vi "NV40.vi"(4 "Position":dbl, 5 "error in (no error)":errorcluster, 6 "Timeout":u32=100, 7 "VISA resource name":refnum<visa-resource-name>, 8 "Command":T1(ring)) -> (0 "error out":errorcluster, 3 "Position out":dbl)   [LabVIEW 2015]
uses:
  <vilib>/Instr/_visa.llb/VISA Open Access Mode.ctl
  <vilib>/Instr/_visa.llb/VISA Configure Serial Port (Instr).vi
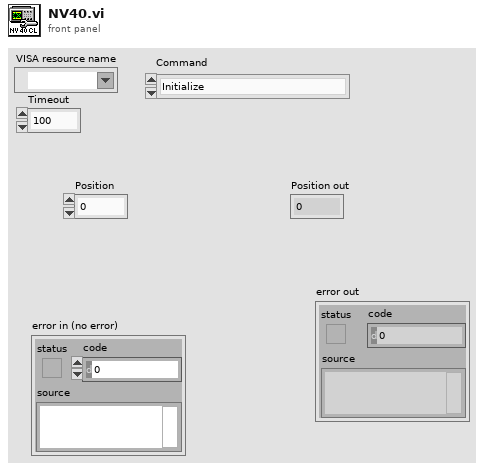
[diagram p1: front panel]
types:
  T1 = enum16{"Initialize", "Close", "Set position", "Get position", "Closed loop on", "Closed loop off", "Remote control on", "Remote control off"}
  T2 = typedef "VISA Open Access Mode.ctl" = u32
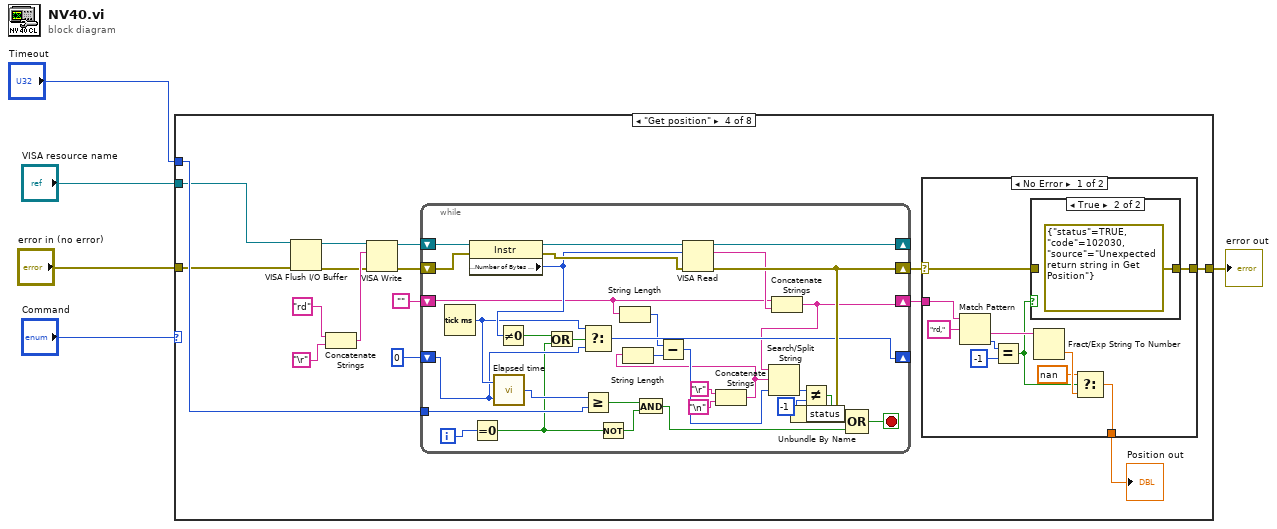
[diagram p0: block diagram]
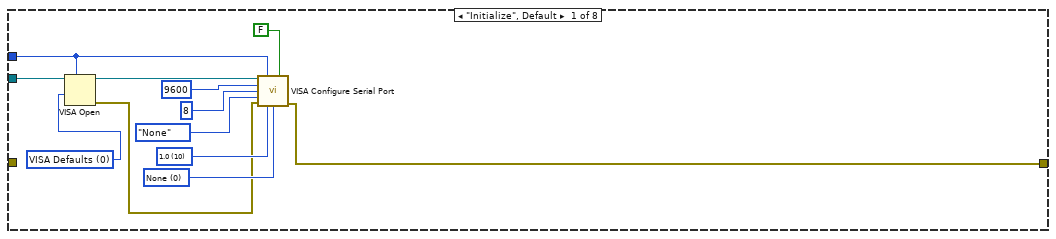
[diagram p2: hidden frame]
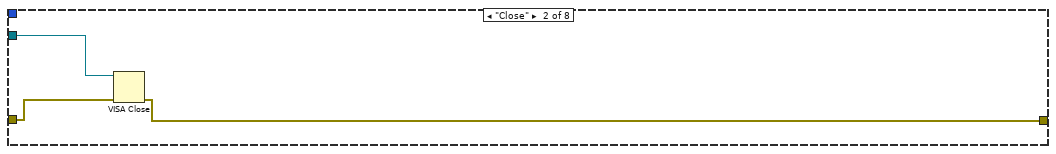
[diagram p3: hidden frame]
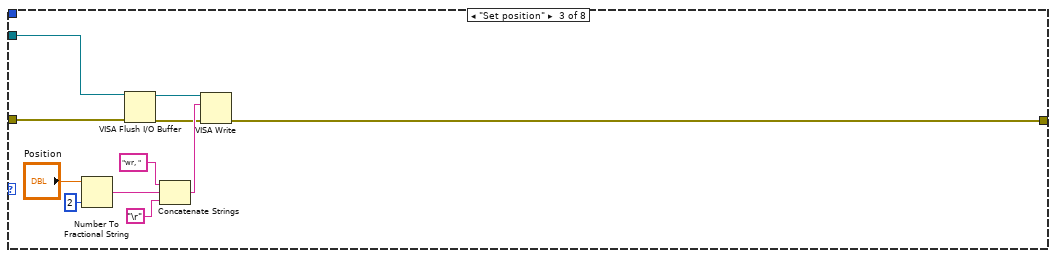
[diagram p4: hidden frame]
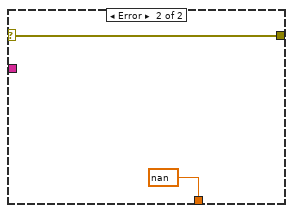
[diagram p6: hidden frame]
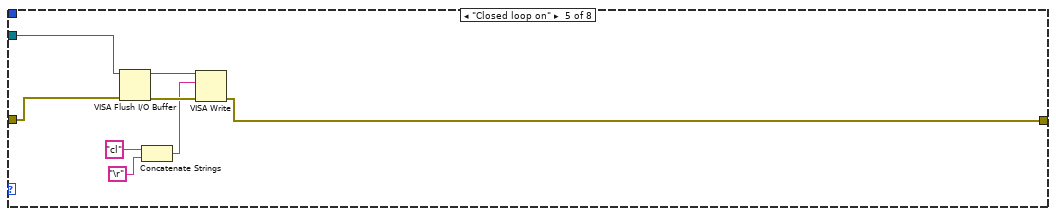
[diagram p7: hidden frame]
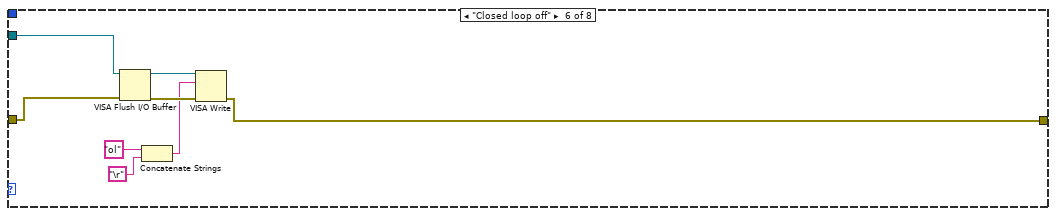
[diagram p8: hidden frame]
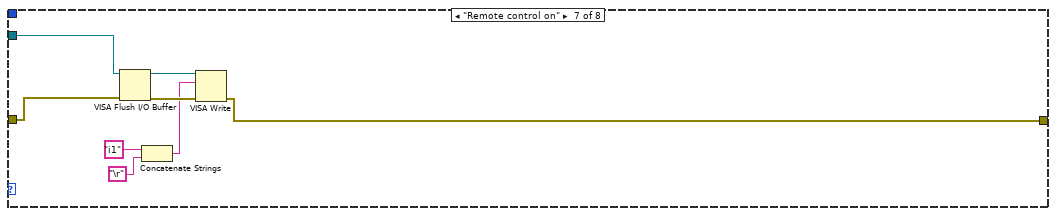
[diagram p9: hidden frame]
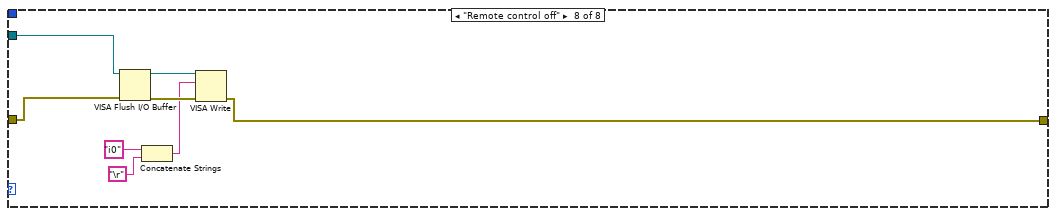
[diagram p10: hidden frame]
diagram:
  n1 = case shown="\"Get position\"" "Command" {
    tunnel: [w6 w18 w25 w33 w99 w107 w115 w123] -> w5
    tunnel: "Timeout" -> [w9 _ _ w39 _ _ _ _]
    tunnel: "VISA resource name" -> [w11 w20 w27 w38 w101 w109 w117 w125]
    tunnel: "error in (no error)" -> [_ w19 w26 w37 w100 w108 w116 w124]
    frame "Initialize", Default {
      w8 = T2 0 items=["VISA Defaults"=0, "Exclusive Lock"=1, "Load Configured Settings"=4] ("Access Mode")
      w12 = u16 0 items=["None", "XON/XOFF", "RTS/CTS", "XON/XOFF & RTS/CTS", "DTR/DSR", "XON/XOFF & DTR/DSR"] ("flow control (0:none)")
      w13 = u16 10 items=["1.0"=10, "1.5"=15, "2.0"=20] ("stop bits (10: 1 bit)")
      n2 = VISA Open(timeout (0)=w9, access mode=w8, VISA resource name=w11) -> (VISA resource name=w10:refnum<visa-resource-name>, error out=w7:errorcluster)  [unwired: 2 in]
      n3 = call-poly "VISA Configure Serial Port"("VISA resource name"=w10, "timeout (10sec)"=w9, "Enable Termination\nChar (T)"=FALSE ("Enable Termination\nChar (T)"), "baud rate (9600)"=u32 9600, "data bits (8)"=u16 8, "parity (0:none)"=enum16{"None", "Odd", "Even", "Mark", "Space"}."None", "error in (no error)"=w7, "stop bits (10: 1 bit)"=w13, "flow control (0:none)"=w12) -> ("error out"=w6:errorcluster)  [unwired: 5 in, 1 out]
    }
    frame "Close" {
      n4 = VISA Close(VISA resource name=w20, error in (no error)=w19) -> (error out=w18:errorcluster)
    }
    frame "Set position" {
      n5 = Number To Fractional String(number="Position", precision (6)=i16 2) -> (F-format string=w21:string)  [unwired: 2 in]
      n6 = VISA Flush I/O Buffer(VISA resource name=w27, error in (no error)=w26) -> (VISA resource name out=w30:refnum<visa-resource-name>, error out=w28:errorcluster)  [unwired: 1 in]
      n7 = Concatenate Strings("wr, ", w21, "\r") -> (w29:string)
      n8 = VISA Write(VISA resource name=w30, write buffer=w29, error in (no error)=w28) -> (error out=w25:errorcluster)  [unwired: 2 out]
    }
    frame "Get position" {
      n9 = VISA Flush I/O Buffer(VISA resource name=w38, error in (no error)=w37) -> (VISA resource name out=w46:refnum<visa-resource-name>, error out=w44:errorcluster)  [unwired: 1 in]
      n10 = Concatenate Strings("rd", "\r") -> (w45:string)
      n11 = VISA Write(VISA resource name=w46, write buffer=w45, error in (no error)=w44) -> (VISA resource name out=w43:refnum<visa-resource-name>, error out=w42:errorcluster)  [unwired: 1 out]
      n12 = while {
        shift-right: [w91] -> _
        shift-left: w43 -> [w95]
        shift-right: [w89] -> w34
        shift-left: w42 -> [w94]
        shift-right: [w71] -> w35
        shift-left: "" -> [w70]
        shift-right: [w79] -> _
        shift-left: u32 0 -> [w76]
        tunnel: w39 -> [w77]
        i -> [w82]
        stop <- w90 stop-if-true
        n13 = Tick Count (ms)() -> (millisecond timer value=w80:u32)
        n14 = property class="Instr"(reference=w95, error in=w94) -> (reference out=w93:refnum<visa-resource-name>, error out=w92:errorcluster, "Serial Settings:Number of Bytes at Serial Port"=w84:u32)
        n15 = Equal To 0?(x=w82) -> (x = 0?=w72:bool)
        n16 = call "Elapsed time.vi"("Start time (ms)"=w76, "Current time (ms)"=w80) -> ("Elapsed time"=w78:u32)
        n17 = Not Equal To 0?(x=w84) -> (x != 0?=w83:bool)
        n18 = Or(x=w83, y=w72) -> (x .or. y?=w81:bool)
        n19 = Select(t=w80, s=w81, f=w76) -> (s? t:f=w79:u32)
        n20 = Greater Or Equal?(x=w78, y=w77) -> (x >= y?=w74:bool)
        n21 = Not(x=w72) -> (.not. x?=w73:bool)
        n22 = String Length(string=w70) -> (length=w68:i32)
        n23 = And(x=w74, y=w73) -> (x .and. y?=w75:bool)
        n24 = VISA Read(VISA resource name=w93, byte count=w84, error in (no error)=w92) -> (VISA resource name out=w91:refnum<visa-resource-name>, read buffer=w88:string, error out=w89:errorcluster)  [unwired: 1 out]
        n25 = Concatenate Strings("\r", "\n") -> (w64:string)
        n26 = String Length(string=w64) -> (length=w69:i32)
        n27 = Subtract(x=w68, y=w69) -> (x-y=w67:i32)
        n28 = Concatenate Strings(w70, w88) -> (w71:string)
        n29 = Search/Split String(string=w71, search string/char (-)=w64, offset (0)=w67) -> (offset of match=w87:i32)  [unwired: 2 out]
        n30 = Unbundle By Name(w89) -> ("status"=w63:bool)
        n31 = Not Equal?(x=w87, y=-1) -> (x != y?=w85:bool)
        n32 = Compound Arithmetic op=OR(w63, w85, w75) -> (w90:bool)
      }
      n33 = case shown="No Error" w34 {
        selector: w34 -> [w52 w62]
        tunnel: w35 -> [w58 _]
        tunnel: [w53 w62] -> w33
        tunnel: [w51 nan] -> w32
        frame No Error {
          n34 = Match Pattern(string=w58, regular expression="rd,") -> (after substring=w56:string, offset past match=w55:i32)  [unwired: 1 in, 2 out]
          n35 = Equal?(x=w55, y=-1) -> (x = y?=w49:bool)
          n36 = case shown="True" w49 {
            tunnel: [w59 errorcluster {"status"=TRUE, "code"=102030, "source"="Unexpected return string in Get Position"} ("error IO")] -> w53
            tunnel: w52 -> [w59 _]
            frame False {
            }
            frame True {
            }
          }
          n37 = Fract/Exp String To Number(string=w56) -> (number=w50:dbl)  [unwired: 3 in, 1 out]
          n38 = Select(t=nan, s=w49, f=w50) -> (s? t:f=w51:dbl)
        }
        frame Error {
        }
      }
      "Position out" <- w32
    }
    frame "Closed loop on" {
      n39 = VISA Flush I/O Buffer(VISA resource name=w101, error in (no error)=w100) -> (VISA resource name out=w103:refnum<visa-resource-name>, error out=w102:errorcluster)  [unwired: 1 in]
      n40 = Concatenate Strings("cl" ("string"), "\r") -> (w98:string)
      n41 = VISA Write(VISA resource name=w103, write buffer=w98, error in (no error)=w102) -> (error out=w99:errorcluster)  [unwired: 2 out]
    }
    frame "Closed loop off" {
      n42 = VISA Flush I/O Buffer(VISA resource name=w109, error in (no error)=w108) -> (VISA resource name out=w111:refnum<visa-resource-name>, error out=w110:errorcluster)  [unwired: 1 in]
      n43 = Concatenate Strings("ol" ("string"), "\r") -> (w106:string)
      n44 = VISA Write(VISA resource name=w111, write buffer=w106, error in (no error)=w110) -> (error out=w107:errorcluster)  [unwired: 2 out]
    }
    frame "Remote control on" {
      n45 = VISA Flush I/O Buffer(VISA resource name=w117, error in (no error)=w116) -> (VISA resource name out=w119:refnum<visa-resource-name>, error out=w118:errorcluster)  [unwired: 1 in]
      n46 = Concatenate Strings("i1" ("string"), "\r") -> (w114:string)
      n47 = VISA Write(VISA resource name=w119, write buffer=w114, error in (no error)=w118) -> (error out=w115:errorcluster)  [unwired: 2 out]
    }
    frame "Remote control off" {
      n48 = VISA Flush I/O Buffer(VISA resource name=w125, error in (no error)=w124) -> (VISA resource name out=w127:refnum<visa-resource-name>, error out=w126:errorcluster)  [unwired: 1 in]
      n49 = Concatenate Strings("i0" ("string"), "\r") -> (w122:string)
      n50 = VISA Write(VISA resource name=w127, write buffer=w122, error in (no error)=w126) -> (error out=w123:errorcluster)  [unwired: 2 out]
    }
  }
  "error out" <- w5
